vi "参数转id.vi"(11 "table":string) -> (3 "id":u16)   [LabVIEW 2016, in "斯坦道氨氮.lvlib"]
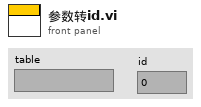
[diagram p1: front panel]
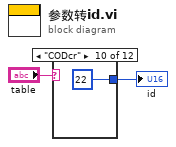
[diagram p0: block diagram]
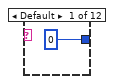
[diagram p2: hidden frame]
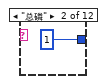
[diagram p3: hidden frame]
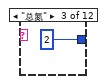
[diagram p4: hidden frame]
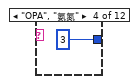
[diagram p5: hidden frame]
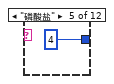
[diagram p6: hidden frame]
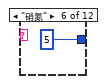
[diagram p7: hidden frame]
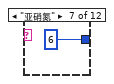
[diagram p8: hidden frame]
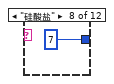
[diagram p9: hidden frame]
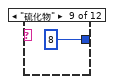
[diagram p10: hidden frame]
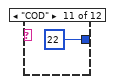
[diagram p11: hidden frame]
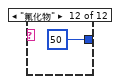
[diagram p12: hidden frame]
diagram:
  n1 = case shown="\"CODcr\"" "table" {
    tunnel: [u16 0 ("id") u16 1 ("id") u16 2 ("id") u16 3 ("id") u16 4 ("id") u16 5 ("id") u16 6 ("id") u16 7 ("id") u16 8 ("id") u16 22 ("id") u16 22 ("id") u16 50 ("id")] -> w1
    frame Default {
    }
    frame "总磷" {
    }
    frame "总氮" {
    }
    frame "OPA", "氨氮" {
    }
    frame "磷酸盐" {
    }
    frame "硝氮" {
    }
    frame "亚硝氮" {
    }
    frame "硅酸盐" {
    }
    frame "硫化物" {
    }
    frame "CODcr" {
    }
    frame "COD" {
    }
    frame "氟化物" {
    }
  }
  "id" <- w1
